vi "gu_select_folder_dialog.vi"(7 "Prompt":T1, 8 "error in":errorcluster, 11 "Start Path":T1) -> (0 "error out":errorcluster, 1 "Cancelled":bool, 3 "Encoded Path":T1)   [LabVIEW 2020, in "G-Unicode.lvlib"]
uses:
  G-Unicode.lvlib
  Types/Encoded UTF-8 String.ctl
  Memory/Copy String.vi/4d47babd-4a2d-4eb7-b91b-7e707d692665.vi
  gu_free.vi
  <vilib>/Utility/error.llb/Error Cluster From Error Code.vi
  lib/g_unicode_32.dll
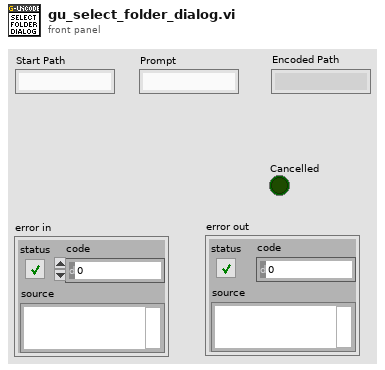
[diagram p1: front panel]
types:
  T1 = typedef "G-Unicode.lvlib/Encoded UTF-8 String.ctl" = string
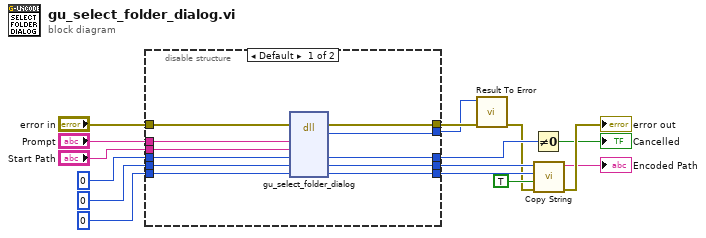
[diagram p0: block diagram]
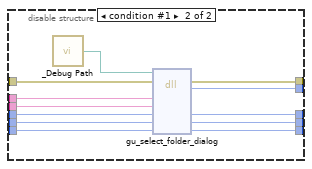
[diagram p2: hidden frame]
diagram:
  n1 = disable-structure shown="Default" {
    disable-tunnel: "error in" -> [w27 w39]
    disable-tunnel: [w26 w38] -> w3
    disable-tunnel: "Prompt" -> [w25 w37]
    disable-tunnel: "Start Path" -> [w24 w36]
    disable-tunnel: i64 0 ("path_pointer") -> [w23 w35]
    disable-tunnel: 0 ("path_length") -> [w22 w34]
    disable-tunnel: [w21 w33] -> w11
    disable-tunnel: [w20 w32] -> w10
    disable-tunnel: [w18 w30] -> w9
    disable-tunnel: 0 ("path_length") -> [w19 w28]
    disable-tunnel: [w17 w29] -> w1
    frame condition #0 (active) {
      n2 = dll-call lib="C:/github/dataflowg/g-unicode/src/LabVIEW/G-Unicode/lib/g_unicode_*.*" fn="gu_select_folder_dialog"(error in=w27, "title"=w25, "default_path"=w24, "cancelled"=w19, "path_pointer"=w23, "path_length"=w22) -> (error out=w26:errorcluster, "result"=w17:i32, "cancelled"=w18:i32, "path_pointer"=w21:i64, "path_length"=w20:i32)  [unwired: 4 in, 1 out]
    }
    frame condition #1 {
      n3 = call "_Debug Path.vi"() -> ("Debug Path"=w31:path)
      n4 = dll-call lib="?" fn="gu_select_folder_dialog"(path in=w31, error in=w39, "title"=w37, "default_path"=w36, "cancelled"=w28, "path_pointer"=w35, "path_length"=w34) -> (error out=w38:errorcluster, "result"=w29:i32, "cancelled"=w30:i32, "path_pointer"=w33:i64, "path_length"=w32:i32)  [unwired: 3 in, 1 out]
    }
  }
  n5 = call "Result To Error.vi"("error in (no error)"=w3, "Result Code"=w1) -> ("error out"=w2:errorcluster)  [unwired: 9 in]
  n6 = Not Equal To 0?(x=w9) -> (x != 0?=→"Cancelled":bool)
  n7 = call "Copy String.vi"("error in"=w2, "free (F)"=TRUE, "size"=w10, "pointer"=w11) -> ("error out"=→"error out":errorcluster, "string"=→"Encoded Path":string)  [unwired: 6 in]
